vi "Homing.vi"(6 "Axis Index":i32, 7 "Motion Parameters":T1={"Timeout"=-1.0, "Blend Mode"=10551335, "Acceleration"=4.0, "Deceleration"=4.0, "Accel. Jerk"=4.0, "Decel. Jerk"=4.0, "Smoothing"=0.5, "Last Blend"=FALSE, "Blend Delay"=-1.0} {"Blend Delay" format="%#_13g"; "Smoothing" format="%#_13g"; "Decel. Jerk" format="%#_13g"; "Accel. Jerk" format="%#_13g"; "Deceleration" format="%#_13g"; "Acceleration" format="%#_13g"; "Blend Mode" items=["At Profile Complete"=10551335, "At Deceleration"=10551334, "After Delay"=10551336]}, 8 "Error In":errorcluster, 9 "Approach  Velocity":dbl=1.0, 10 "Search Velocity":dbl=2.0, 11 "Axis Reference In":refnum<k21>="Z Axis") -> (0 "Error Out":errorcluster, 3 "Axis Reference Out":refnum<k21>="Z Axis")   [LabVIEW 2018]
doc: "Homes the axis to the Reverse Limit."
uses:
  Type Defs/The Motion Parameters.ctl
  <vilib>/Motion/Express/_s/nimc.ex.findReferenceMove.startReferenceMove.axis.modeReverseLimit.vi
  <vilib>/Motion/Express/_s/nimc.ex.resetPosition.resetPosition.axis.vi
  <vilib>/Motion/BlockNode/FB.NIMotion.xnode
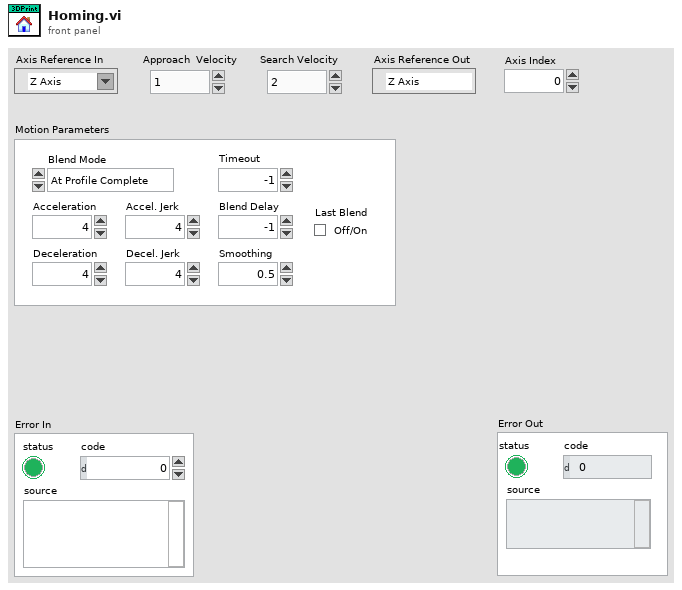
[diagram p1: front panel]
types:
  T1 = typedef "The Motion Parameters.ctl" = cluster{"Timeout":dbl, "Blend Mode":i32, "Acceleration":dbl, "Deceleration":dbl, "Accel. Jerk":dbl, "Decel. Jerk":dbl, "Smoothing":dbl, "Last Blend":bool, "Blend Delay":dbl}
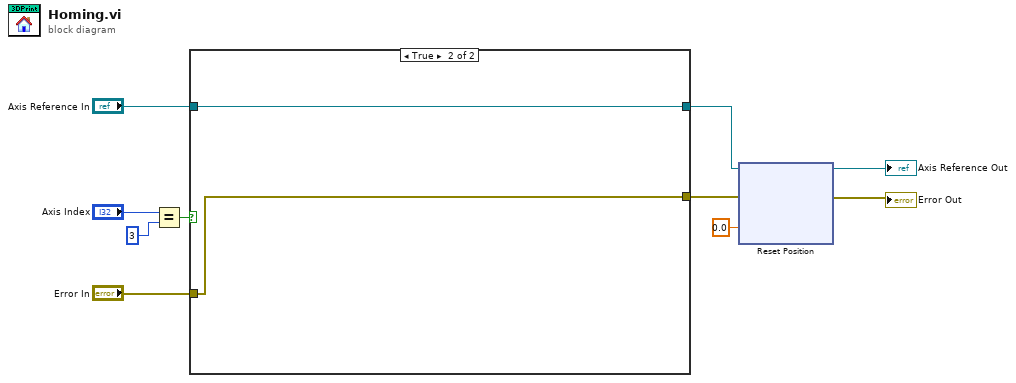
[diagram p0: block diagram]
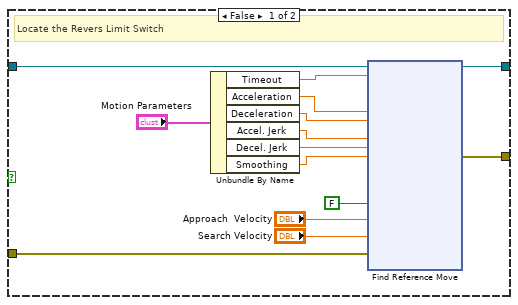
[diagram p2: hidden frame]
diagram:
  n1 = Equal?(x="Axis Index", y=3) -> (x = y?=w3:bool)
  n2 = case shown="True" w3 {
    tunnel: "Error In" -> [w24 w44]
    tunnel: "Axis Reference In" -> [w13 w43]
    tunnel: [w12 w43] -> w8
    tunnel: [w11 w44] -> w5
    frame False {
      # "Locate the Revers Limit Switch"
      n3 = Unbundle By Name("Motion Parameters") -> ("Timeout"=w14:dbl, "Acceleration"=w15:dbl, "Deceleration"=w16:dbl, "Accel. Jerk"=w17:dbl, "Decel. Jerk"=w18:dbl, "Smoothing"=w19:dbl)
      n4 = xnode "Find Reference Move"("approach forward"=FALSE, "approach velocity"="Approach  Velocity", "search velocity"="Search Velocity", "error in"=w24, "resource"=w13, "timeout"=w14, "acceleration"=w15, "deceleration"=w16, "accel. jerk"=w17, "decel. jerk"=w18, "smoothing"=w19) -> ("resource out"=w12:refnum<k21>, "error out"=w11:errorcluster)  [unwired: 1 out]
    }
    frame True {
    }
  }
  n5 = xnode ("Reset Position")("position"=0.0, "resource"=w8, "error in"=w5) -> ("resource out"=→"Axis Reference Out":refnum<k21>, "error out"=→"Error Out":errorcluster)
